vi "read_z_voltage.vi"(8 "error in":errorcluster, 11 "PZT in":refnum<class "PZT.lvclass">) -> (0 "error out":errorcluster, 2 "Z Voltage out":i16, 3 "PZT out":refnum<class "PZT.lvclass">)   [LabVIEW 2020, in "PZT.lvclass"]
uses:
  PZT.lvclass
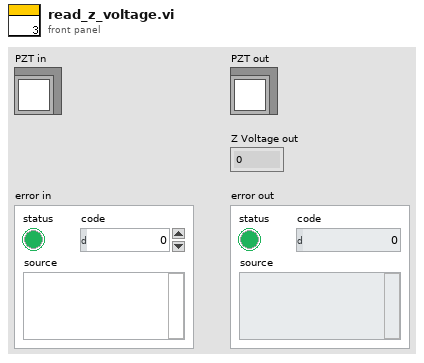
[diagram p1: front panel]
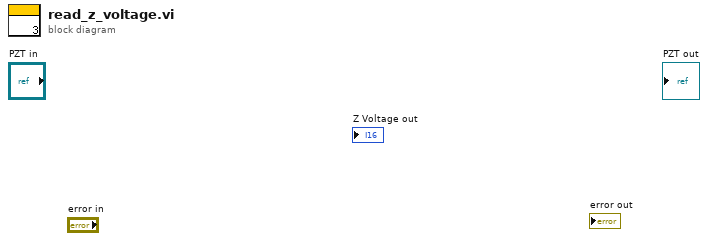
[diagram p0: block diagram]
diagram:
